vi "Filter Errors.vi"(8 "error in (no error)":errorcluster, 10 "Errors to filter":i32[](array[numeric]), 11 "Local Error Manager in":refnum<class "Local Error Manager.lvclass">) -> (0 "error out":errorcluster, 2 "Filters to remove":set{i32}(c389), 3 "Local Error Manager out":refnum<class "Local Error Manager.lvclass">)   [LabVIEW 2026, in "TALOS.lvlib" / "Error Manager.lvlib" / "Local Error Manager.lvclass"]
uses:
  Local Error Manager.lvclass
  Ancestor/Ancestor/Ancestor.lvclass/Ancestor.ctl
  Support VIs/Generate Error.vi
  FGV/Error Memory/Get Error Description.vi
  Support VIs/Get PC name.vi
  Ancestor/Ancestor/Read ID.vi
  Support VIs/Get Class Name.vi
  <vilib>/Utility/error.llb/Clear Errors.vi
  FGV/Error Memory/Error Memory Core.vi
  <vilib>/AdvancedString/Delimited String to 1D String Array.vi
  <vilib>/AdvancedString/Delimited String to 1D String Array (string).vi
  Support VIs/Circus Root Path.vi
  FGV/Error Memory/Error Crt Lvl checker.vi
  FGV/Error Memory/Error Memory Core.vi/40c8088d-b597-4017-91af-faa98e00292e.vi
  FGV/Error Memory/Error Memory Core.vi/d4a3ab98-063c-4e44-b43d-fbdcfe6c2be2.vi
  Support VIs/Global Memory.vi
  <vilib>/Utility/LVClass/Get LV Class Name.vi
  Support VIs/Is in Packed Library.vi
  Support VIs/TALOS Root path.vi
  Support VIs/Read CSV worksheet.vi
  Support VIs/Global Constants.vi
  <vilib>/Utility/error.llb/General Error Handler.vi
  Support VIs/Error Log.vi
  Error Manager.lvclass
  Ancestor/Ancestor/Ancestor.lvclass
  <vilib>/Comparison/Equal/Equal Functor/Equal Functor.lvclass
  Classes/Error Filter/Error Filter.lvclass
  TALOS.lvlib
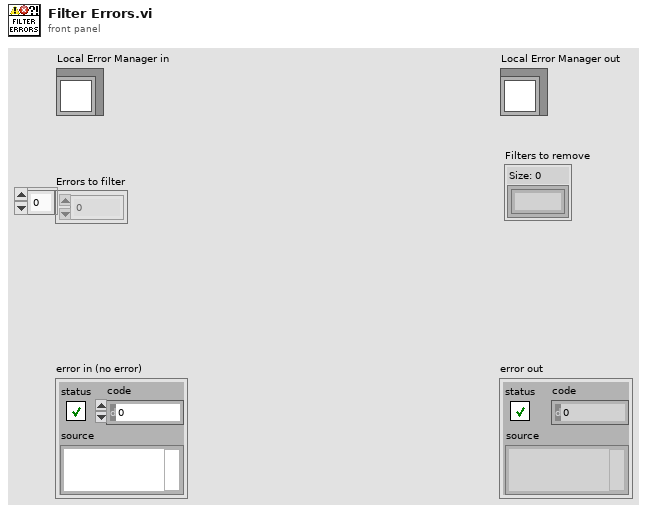
[diagram p1: front panel]
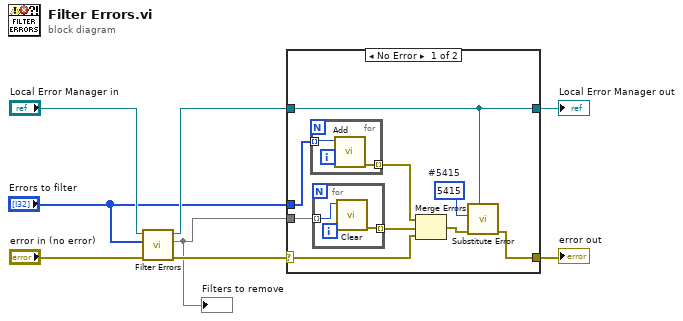
[diagram p0: block diagram]
diagram:
  n1 = call-parent "Filter Errors.vi"("error in (no error)"="error in (no error)", "Errors to filter"="Errors to filter", "Error Manager in"="Local Error Manager in") -> ("error out"=w7:errorcluster, "Filters to remove"=w1:set{i32}, "Error Manager out"=w5:refnum<class "Local Error Manager.lvclass">)  [unwired: 6 in]
  "Filters to remove" <- w1
  n2 = case shown="No Error" w7 {
    selector: w7 -> [w17 w23]
    tunnel: [w14 w23] -> w3
    tunnel: [w13 w22] -> w2
    tunnel: w5 -> [w13 w22]
    tunnel: "Errors to filter" -> [w12 _]
    tunnel: w1 -> [w9 _]
    frame No Error {
      w16 = 5415  # #5415
      n3 = for {
        tunnel: w12 -> [w20] mode=indexing
        tunnel: [w21] -> w10 mode=indexing
        n4 = call "Add.vi"("Error Code"=w20) -> ("error out"=w21:errorcluster)  [unwired: 10 in]
      }
      n5 = for {
        tunnel: [w19] -> w11 mode=indexing
        tunnel: w9 -> [w18] mode=indexing
        n6 = call "Clear.vi"("Error Code"=w18) -> ("error out"=w19:errorcluster)  [unwired: 10 in]
      }
      n7 = Merge Errors(w10, w11, w17) -> (w15:errorcluster)
      n8 = call "Substitute Error.vi"("LabVIEW Object"=w13, "error in (no error)"=w15, "Error Code"=w16) -> ("error out"=w14:errorcluster)  [unwired: 8 in]
    }
    frame Error {
    }
  }
  "error out" <- w3
  "Local Error Manager out" <- w2
